vi "GUI Mode Change.vi"() -> ()   [LabVIEW 2011]
uses:
  Types Definitions/Type TCP State.ctl
  <vilib>/Platform/TimedLoop/XDataNode/timing_clust.ctl
  <vilib>/Platform/TimedLoop/XDataNode/nitl_modes.ctl
  <vilib>/Platform/TimedLoop/XDataNode/wakeup.ctl
  <vilib>/Platform/TimedLoop/XDataNode/XDataNode.xnode
  Type Definitions.lvlib
  LNLS Control VIs.lvlib
  Misc VIs.lvlib
  <vilib>/Platform/TimedLoop/XDataNode/XDNodeRunTimeDep.lvlib
panel:
  in  "Operation Mode":T1(ring)
  out "LNLS Control FOFB Configuration":T2
  in  "Change":bool
  out "error out":errorcluster
  in  "error in (no error)":errorcluster
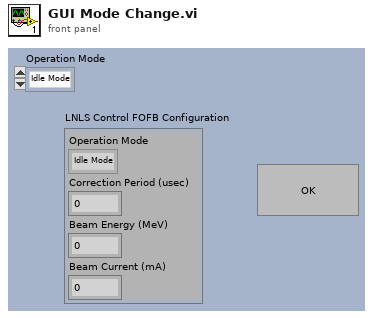
[diagram p1: front panel]
types:
  T1 = enum16{"Idle Mode", "Error Mode", "Manual Mode", "FOFB Mode", "RMM Mode"}
  T2 = cluster{"Operation Mode":enum16{"Idle Mode", "Error Mode", "Manual Mode", "FOFB Mode", "RMM Mode"}, "Correction Period (usec)":i32, "Beam Energy (MeV)":sgl, "Beam Current (mA)":sgl}
  T3 = typedef "Type Definitions.lvlib/Type TCP State.ctl" = enum16{"Idle", "Wait Connection", "Read Data", "Process Data", "Write Data", "Close Connection"}
  T4 = typedef "XDNodeRunTimeDep.lvlib/timing_clust.ctl" = cluster{"Expected End [f-1]":u64, "Actual End [f-1]":u64, "Finished Late? [f-1]":bool, "Expected End [i-1]":u64, "Actual End [i-1]":u64, "Finished Late? [i-1]":bool, "Expected Start [i]":u64, "Actual Start [i]":u64, "Expected Start [f]":u64, "Actual Start [f]":u64, "Source Name":string, "Structure Name":string, "Period":i64, "Deadline":i64, "Offset":i64, "Start":i64, "Priority":i32, "Timeout":i32, "Mode":T5, "Wakeup Reason":T6, "Error":errorcluster, "Source Type":string, "Secondary Source Type":string, "Global End Time":u64, "Global Start Time":u64, "Frame Duration":u64, "Iteration Duration":u64, "Assigned CPU":i32, "I/O Scan Engine Mode":u32}
  T5 = typedef "XDNodeRunTimeDep.lvlib/nitl_modes.ctl" = enum32{"No Change", "Process missed periods, maintain original phase", "Discard missed periods, maintain original phase", "Process missed periods, ignore original phase", "Discard missed periods, ignore original phase"}
  T6 = typedef "XDNodeRunTimeDep.lvlib/wakeup.ctl" = enum32{"Normal", "Aborted", "Asynchronous wakeup", "Timing source error", "Timed loop error", "Timeout"}
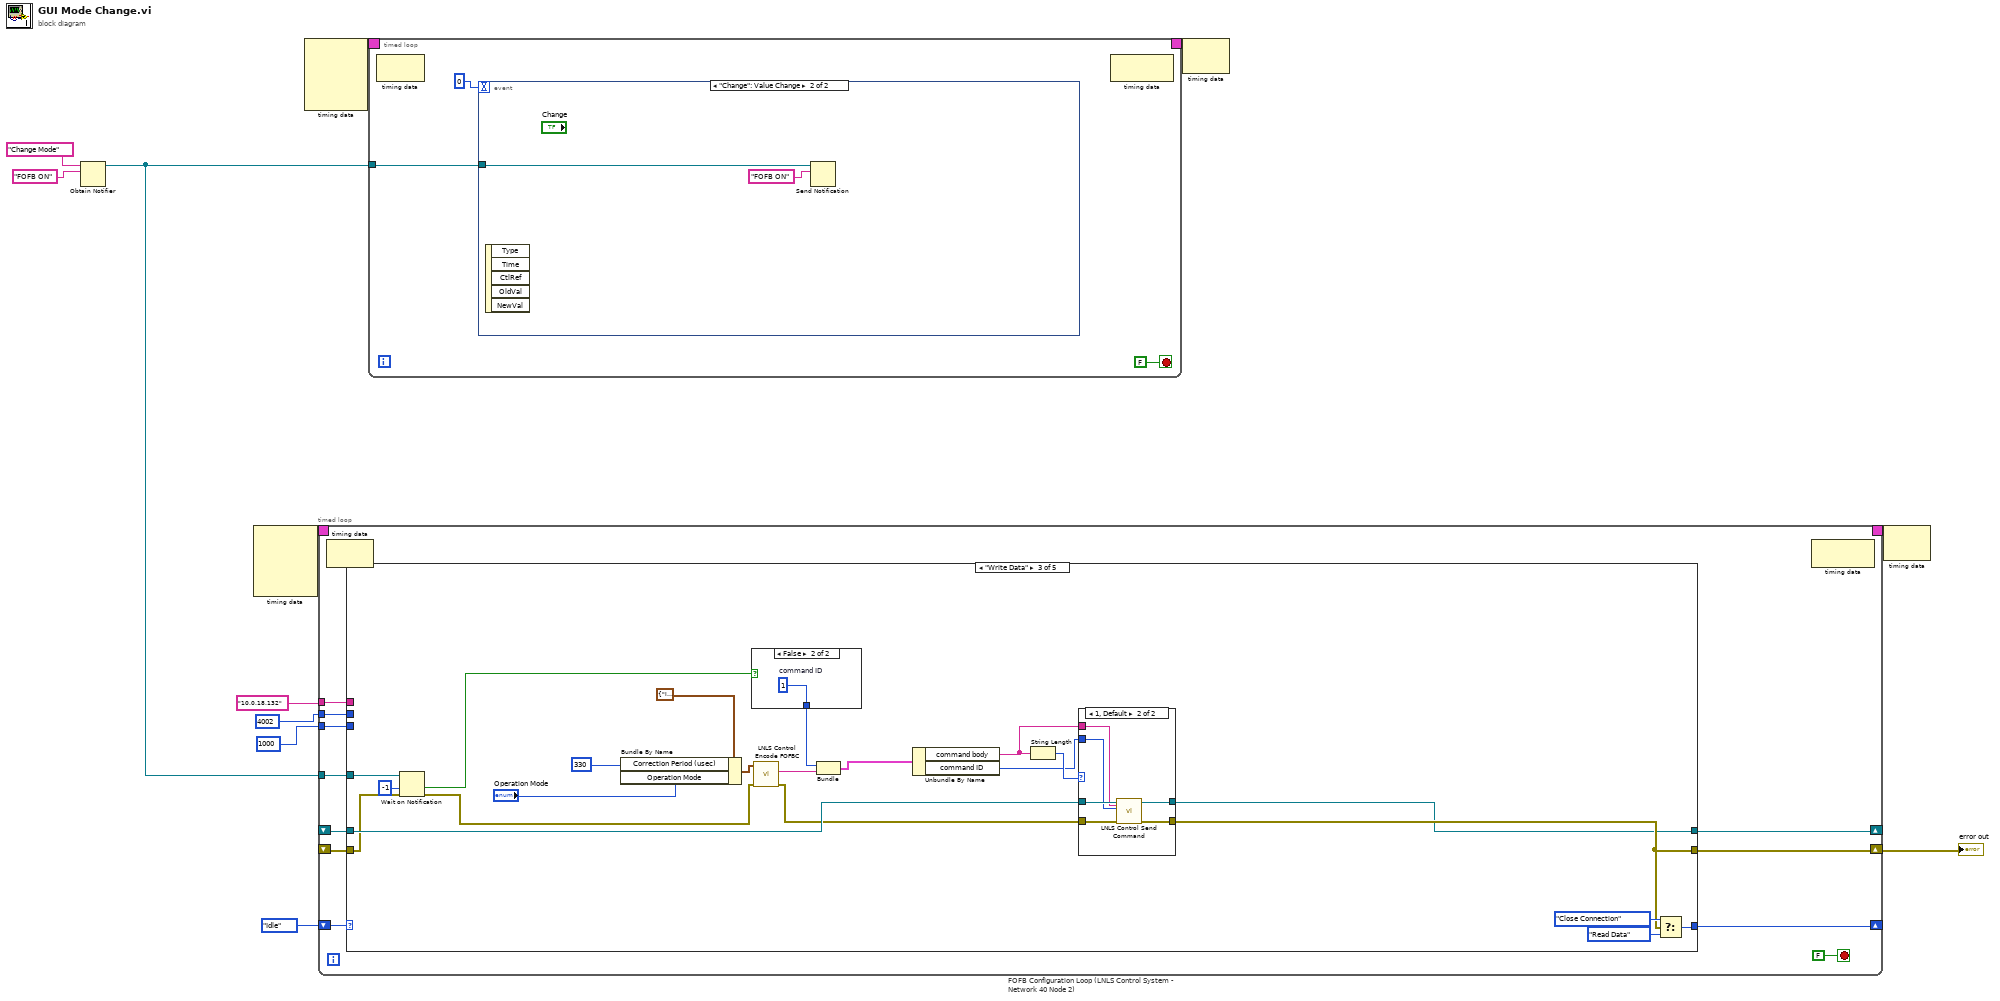
[diagram p0: block diagram]
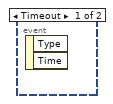
[diagram p2: hidden frame]
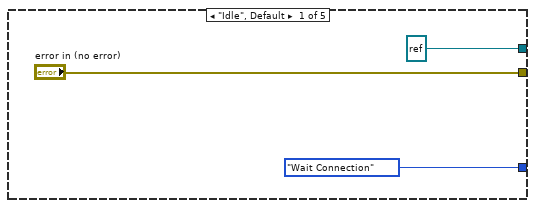
[diagram p3: hidden frame]
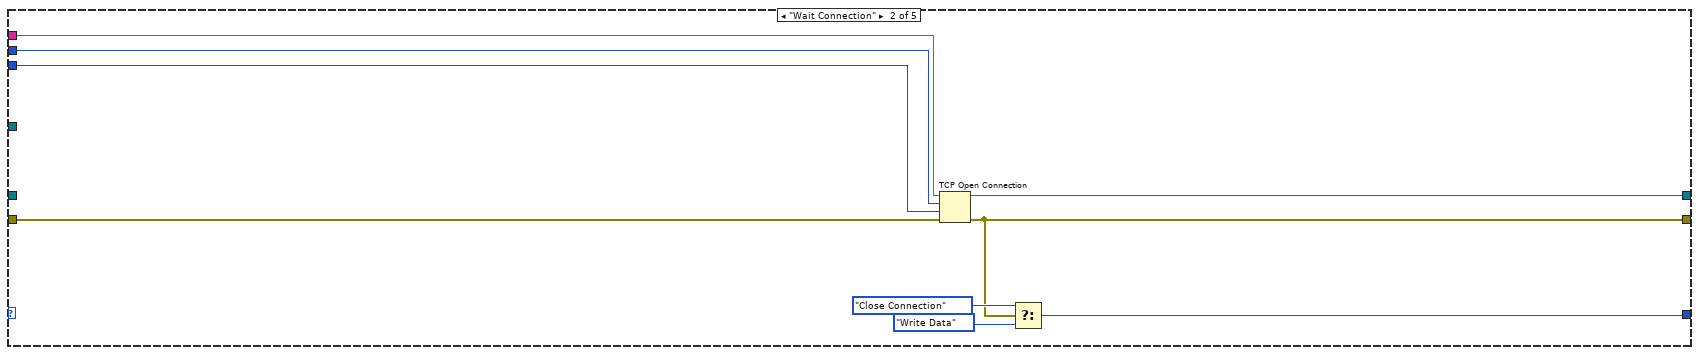
[diagram p4: hidden frame]
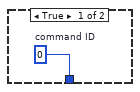
[diagram p5: hidden frame]
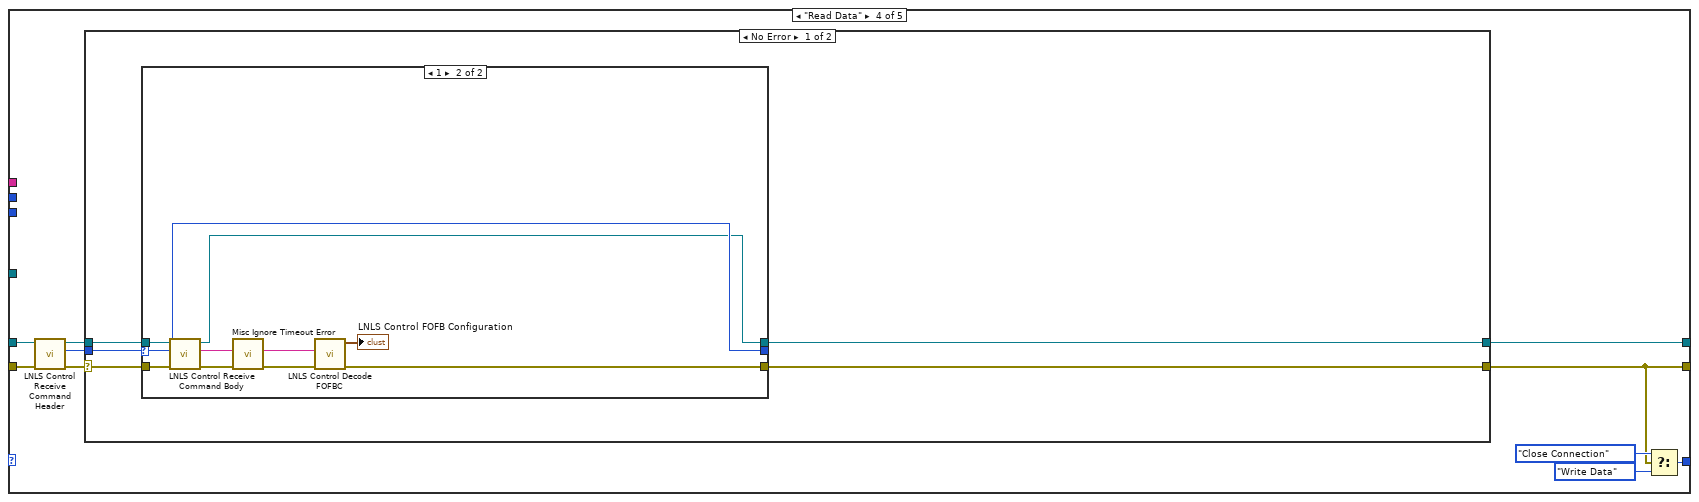
[diagram p7: hidden frame]
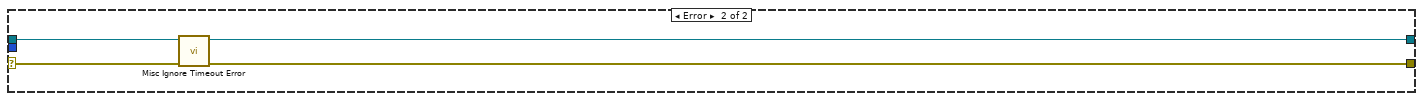
[diagram p9: hidden frame]
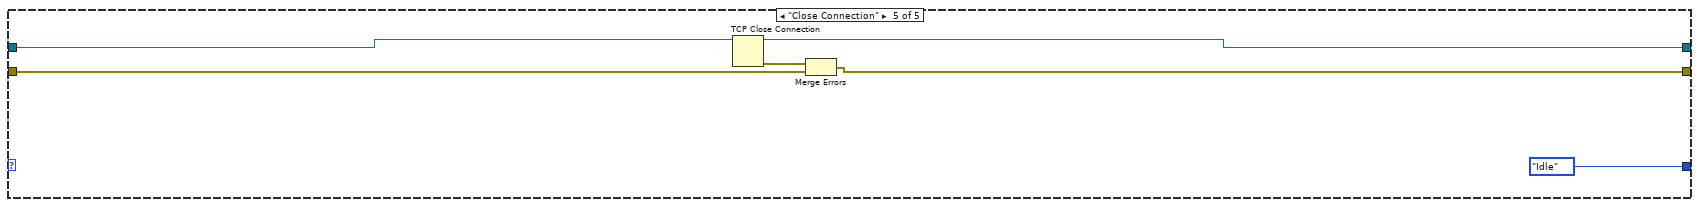
[diagram p10: hidden frame]
diagram:
  n1 = Obtain Notifier(name (unnamed)="Change Mode", notification data type="FOFB ON" ("notification")) -> (notifier out=w2:refnum<notifier>)  [unwired: 2 in, 2 out]
  n2 = node-c288() -> (w12:T4)  [unwired: 4 in]
  n3 = node-c288() -> (w5:T4)  [unwired: 4 in]
  n4 = timed-loop "FOFB Configuration Loop (LNLS Control System - Network 40 Node 2)" {
    shift-right: [w21] -> _
    shift-left: Type_TCP_State."Idle" ("f") -> [w23]
    shift-right: [w22] -> _
    shift-left: _ -> [w20]
    shift-right: [w15] -> w10
    shift-left: _ -> [w19]
    tunnel: "10.0.18.132" ("LNLS Control Network IP") -> [w18]
    tunnel: u16 4002 ("LNLS Control Network FOFB Configuration TCP Port") -> [w17]
    tunnel: 1000 ("TCP Listening Timeout") -> [w16]
    timing: w12 -> [_]
    timing-out: [_] -> w11
    tunnel: w2 -> [w13]
    stop <- FALSE stop-if-true
    n5 = node-c288() -> ()  [unwired: 1 in, 1 out]
    n6 = case shown="\"Write Data\"" w23 {
      tunnel: [refnum<k5> refnum ("connection ID") w34 w51 w79 w104] -> w22
      tunnel: ["error in (no error)" w31 w53 w71 w100] -> w15
      tunnel: [Type_TCP_State."Wait Connection" w37 w57 w78 Type_TCP_State."Idle"] -> w21
      tunnel: w20 -> [_ _ w52 w76 w105]
      tunnel: w19 -> [_ w32 w43 w77 w101]
      tunnel: w18 -> [_ w30 _ _ _]
      tunnel: w17 -> [_ w29 _ _ _]
      tunnel: w16 -> [_ w33 _ _ _]
      tunnel: w13 -> [_ _ w44 _ _]
      frame "Idle", Default {
      }
      frame "Wait Connection" {
        n7 = TCP Open Connection(address=w30, remote port or service name=w29, timeout ms (60000)=w33, error in (no error)=w32) -> (connection ID=w34:refnum<k5>, error out=w31:errorcluster)  [unwired: 1 in]
        n8 = Select(t=Type_TCP_State."Close Connection", s=w31, f=Type_TCP_State."Write Data") -> (s? t:f=w37:T3)
      }
      frame "Write Data" {
        n9 = Wait on Notification(notifier=w44, timeout in ms (-1)=-1, error in (no error)=w43) -> (timed out?=w40:bool, error out=w42:errorcluster)  [unwired: 1 in, 2 out]
        n10 = Bundle By Name(cluster=T2 {"Operation Mode"=enum."Idle Mode", "Correction Period (usec)"=0, "Beam Energy (MeV)"=0.0, "Beam Current (mA)"=0.0} ("LNLS Control FOFB Configuration Out"), "Correction Period (usec)"=u32 330 ("Correction Period"), "Operation Mode"="Operation Mode") -> (w48:T2)
        n11 = case shown="False" w40 {
          tunnel: [w60 w61] -> w49
          frame True {
            w60 = u8 0  # command ID
          }
          frame False {
            w61 = u8 1  # command ID
          }
        }
        n12 = call "LNLS Control Encode FOFBC.vi"("error in (no error)"=w42, "LNLS Control FOFB Configuration"=w48) -> ("error out"=w41:errorcluster, "command body"=w50:string)  [unwired: 8 in]
        n13 = Bundle("command ID"=w49, "command body"=w50) -> (w45:cluster{"command ID":u8, "command body":string})  [unwired: 1 in]
        n14 = Unbundle By Name(w45) -> ("command body"=w56:string, "command ID"=w54:u8)
        n15 = String Length(string=w56) -> (length=w55:i32)
        n16 = case shown="1, Default" w55 {
          tunnel: w52 -> [w62 w69]
          tunnel: w41 -> [w63 w68]
          tunnel: [w63 w67] -> w53
          tunnel: [w62 w66] -> w51
          tunnel: w56 -> [_ w65]
          tunnel: w54 -> [_ w64]
          frame 0 {
          }
          frame 1, Default {
            n17 = call "LNLS Control Send Command.vi"("command body"=w65, "error in (no error)"=w68, "command ID"=w64, "connection ID"=w69) -> ("error out"=w67:errorcluster, "connection ID out"=w66:refnum<k5>)  [unwired: 6 in]
          }
        }
        n18 = Select(t=Type_TCP_State."Close Connection", s=w53, f=Type_TCP_State."Read Data") -> (s? t:f=w57:T3)
      }
      frame "Read Data" {
        n19 = call "LNLS Control Receive Command Header.vi"("error in (no error)"=w77, "connection ID"=w76) -> ("error out"=w73:errorcluster, "command ID"=w70:u8, "connection ID out"=w75:refnum<k5>)  [unwired: 7 in]
        n20 = case shown="No Error" w73 {
          selector: w73 -> [w82 w98]
          tunnel: [w81 w99] -> w79
          tunnel: [w80 w97] -> w71
          tunnel: w75 -> [w84 w99]
          tunnel: w70 -> [w83 _]
          frame No Error {
            n21 = case shown="1" w83 {
              selector: w83 -> [w85 w92]
              tunnel: w82 -> [w87 w95]
              tunnel: [w87 w93] -> w80
              tunnel: [w86 w91] -> w81
              tunnel: w84 -> [w86 w96]
              tunnel: [w85 w92] -> _
              frame 0, Default {
              }
              frame 1 {
                n22 = call "LNLS Control Receive Command Body.vi"("error in (no error)"=w95, "connection ID"=w96) -> ("error out"=w90:errorcluster, "command body"=w94:string, "connection ID out"=w91:refnum<k5>)  [unwired: 6 in, 1 out]
                n23 = call "Misc Ignore Timeout Error.vi"("error in (no error)"=w90) -> ("error out"=w89:errorcluster)  [unwired: 10 in]
                n24 = call "LNLS Control Decode FOFBC.vi"("error in (no error)"=w89, "command body"=w94) -> ("error out"=w93:errorcluster, "LNLS Control FOFB Configuration"=→"LNLS Control FOFB Configuration":T2)  [unwired: 8 in]
              }
            }
          }
          frame Error {
            n25 = call "Misc Ignore Timeout Error.vi"("error in (no error)"=w98) -> ("error out"=w97:errorcluster)  [unwired: 10 in]
          }
        }
        n26 = Select(t=Type_TCP_State."Close Connection", s=w71, f=Type_TCP_State."Write Data") -> (s? t:f=w78:T3)
      }
      frame "Close Connection" {
        n27 = TCP Close Connection(connection ID=w105) -> (connection ID out=w104:refnum<k5>, error out=w102:errorcluster)  [unwired: 2 in]
        n28 = Merge Errors(w102, w101) -> (w100:errorcluster)
      }
    }
    n29 = node-c288() -> ()  [unwired: 1 in, 1 out]
  }
  "error out" <- w10
  n30 = timed-loop {
    timing: w5 -> [_]
    timing-out: [_] -> w4
    tunnel: w2 -> [w107]
    stop <- FALSE stop-if-true
    n31 = node-c288() -> ()  [unwired: 1 in, 1 out]
    n32 = event shown="[1] \"Change\": Value Change" {
      selector: _ -> [_ _]
      dyn-events: _ -> [_ _]
      timeout: 0 -> [_ _]
      tunnel: w107 -> [_ w110]
      event Timeout {
        n33 = event-data() -> ()  [unwired: 1 in, 2 out]
      }
      event "Change": Value Change {
        n34 = event-data() -> ()  [unwired: 1 in, 5 out]
        n35 = Send Notification(notification="FOFB ON", notifier=w110) -> ()  [unwired: 1 in, 2 out]
      }
    }
    n36 = node-c288() -> ()  [unwired: 1 in, 1 out]
  }
  n37 = node-c288(w4) -> ()  [unwired: 1 out]
  n38 = node-c288(w11) -> ()  [unwired: 1 out]
